vi "Lift_LabVIEW.vi"() -> ()   [LabVIEW 2019]
panel:
  out "Door_Closed":bool
  out "Door_Open":bool
  out "Count":i32
  out "Lift2":bool
  in  "Close":bool
  in  "Open":bool
  out "?":bool
  out "?":bool
  out "?":bool
  out "Target_Pos":i32
  in  "FLOOR_1_DN":bool
  in  "FLOOR_3_UP":bool
  in  "FLOOR_2_DN":bool
  in  "FLOOR_2_UP":bool
  out "Current_Pos":i32
  out "Up/Down":bool
  out "On/Off":bool
  out "Lift":bool
  in  "stop":bool
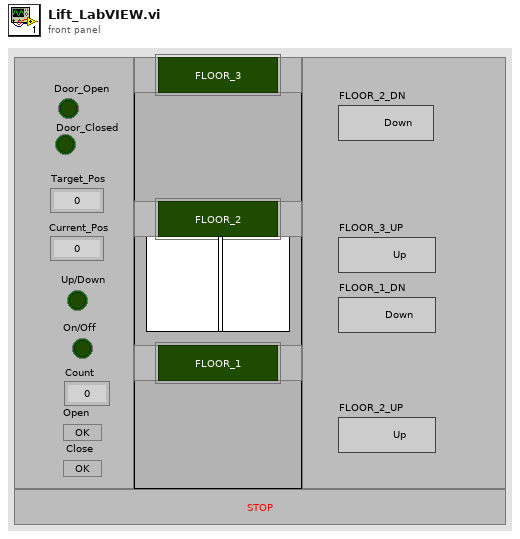
[diagram p1: front panel]
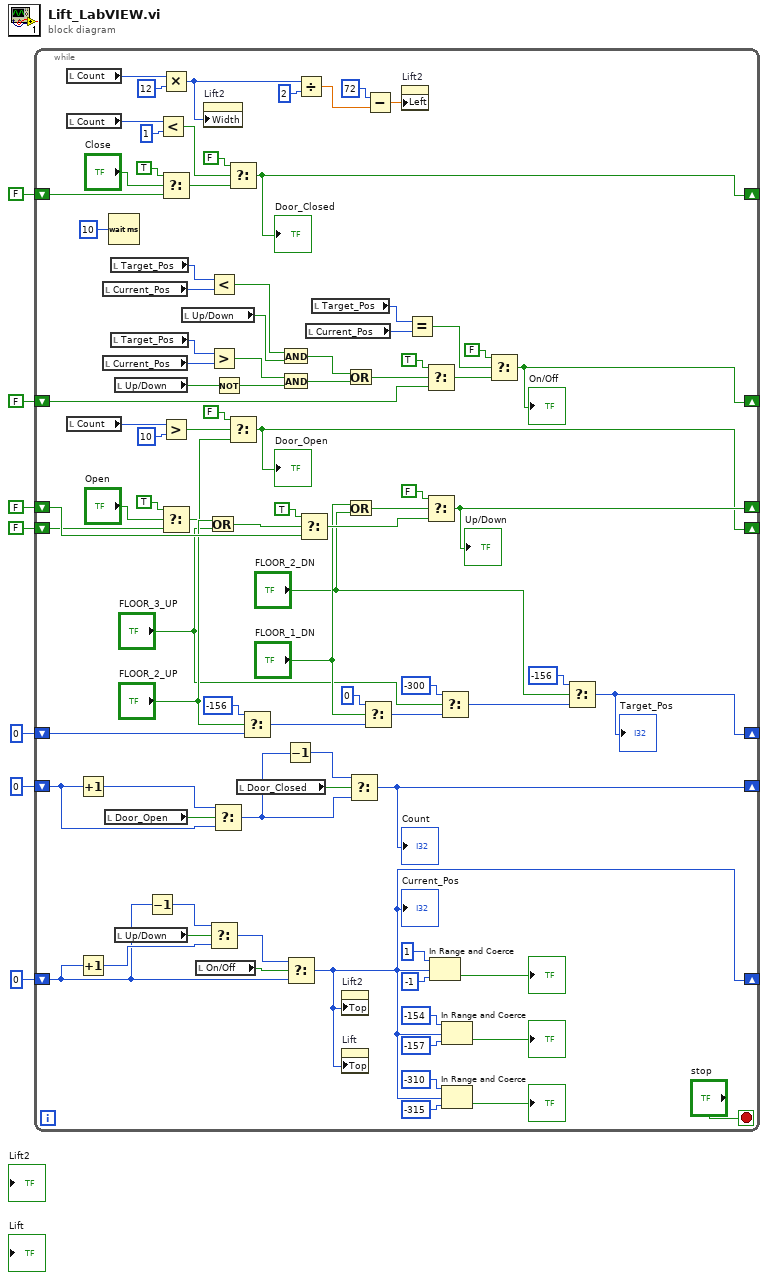
[diagram p0: block diagram]
diagram:
  n1 = while {
    shift-right: [w93] -> _
    shift-left: FALSE -> [w97]
    shift-right: [w8] -> _
    shift-left: 0 -> [w80]
    shift-right: [w84] -> _
    shift-left: FALSE -> [w86]
    shift-right: [w79] -> _
    shift-left: 0 -> [w78]
    shift-right: [w36] -> _
    shift-left: 0 -> [w40]
    shift-right: [w29] -> _
    shift-left: FALSE -> [w32]
    shift-right: [w25] -> _
    shift-left: FALSE -> [w27]
    stop <- "stop" stop-if-true
    n2 = local read "Count"() -> (w15:i32)
    n3 = local read "Count"() -> (w20:i32)
    n4 = local read "Count"() -> (w23:i32)
    n5 = Increment(x=w40) -> (x+1=w38:i32)
    n6 = Increment(x=w80) -> (x+1=w90:i32)
    n7 = local read "Current_Pos"() -> (w64:i32)
    n8 = local read "Current_Pos"() -> (w50:i32)
    n9 = local read "Door_Open"() -> (w17:bool)
    n10 = Wait (ms)(milliseconds to wait=u32 10) -> ()  [unwired: 1 out]
    n11 = local read "Target_Pos"() -> (w65:i32)
    n12 = local read "Target_Pos"() -> (w51:i32)
    n13 = local read "Up/Down"() -> (w54:bool)
    n14 = local read "Up/Down"() -> (w81:bool)
    n15 = Decrement(x=w80) -> (x-1=w91:i32)
    n16 = Less?(x=w20, y=1) -> (x < y?=w18:bool)
    n17 = Multiply(x=w15, y=12) -> (x*y=w12:i32)
    n18 = Select(t=TRUE, s="Close", f=w27) -> (s? t:f=w28:bool)
    n19 = Greater?(x=w23, y=10) -> (0:w21:bool)
    n20 = Select(t=TRUE, s="Open", f=w32) -> (s? t:f=w33:bool)
    n21 = local read "Up/Down"() -> (w62:bool)
    n22 = local read "On/Off"() -> (w88:bool)
    n23 = property on="Lift2" class="Bool (strict)"("Width"=w12) -> ()  [unwired: 2 in, 2 out]
    n24 = Or(x="FLOOR_2_UP", y="FLOOR_3_UP") -> (x .or. y?=w69:bool)
    n25 = Less?(x=w65, y=w64) -> (x < y?=w63:bool)
    n26 = Greater?(x=w51, y=w50) -> (0:w57:bool)
    n27 = Select(t=w91, s=w81, f=w90) -> (s? t:f=w89:i32)
    n28 = Select(t=w38, s=w17, f=w40) -> (s? t:f=w39:i32)
    n29 = Not(x=w54) -> (.not. x?=w55:bool)
    n30 = Select(t=FALSE, s=w18, f=w28) -> (s? t:f=w25:bool)
    "Door_Closed" <- w25
    n31 = Select(t=FALSE, s=w21, f=w33) -> (s? t:f=w29:bool)
    "Door_Open" <- w29
    n32 = local read "Door_Closed"() -> (w16:bool)
    n33 = Select(t=-156, s="FLOOR_2_UP", f=w78) -> (s? t:f=w77:i32)
    n34 = And(x=w63, y=w62) -> (x .and. y?=w61:bool)
    n35 = And(x=w57, y=w55) -> (x .and. y?=w52:bool)
    n36 = Decrement(x=w39) -> (x-1=w37:i32)
    n37 = Select(t=w89, s=w88, f=w80) -> (s? t:f=w8:i32)
    "Current_Pos" <- w8
    n38 = Divide(x=w12, y=2) -> (x/y=w11:dbl)
    n39 = Select(t=TRUE, s=w69, f=w86) -> (s? t:f=w85:bool)
    n40 = local read "Current_Pos"() -> (w59:i32)
    n41 = local read "Target_Pos"() -> (w60:i32)
    n42 = property on="Lift2" class="Bool (strict)"("Top"=w8) -> ()  [unwired: 2 in, 2 out]
    n43 = property on="Lift" class="Bool (strict)"("Top"=w8) -> ()  [unwired: 2 in, 2 out]
    n44 = Or(x=w61, y=w52) -> (x .or. y?=w53:bool)
    n45 = Or(x="FLOOR_1_DN", y="FLOOR_2_DN") -> (x .or. y?=w66:bool)
    n46 = Select(t=w37, s=w16, f=w39) -> (s? t:f=w36:i32)
    "Count" <- w36
    n47 = Select(t=0, s="FLOOR_1_DN", f=w77) -> (s? t:f=w76:i32)
    n48 = Subtract(x=i16 72, y=w11) -> (x-y=w9:dbl)
    n49 = property on="Lift2" class="Bool (strict)"("Left"=w9) -> ()  [unwired: 2 in, 2 out]
    n50 = Equal?(x=w60, y=w59) -> (x = y?=w58:bool)
    n51 = Select(t=TRUE, s=w53, f=w97) -> (s? t:f=w95:bool)
    n52 = Select(t=FALSE, s=w66, f=w85) -> (s? t:f=w84:bool)
    "Up/Down" <- w84
    n53 = In Range and Coerce(upper limit=1, x=w8, lower limit=-1) -> (In Range?=→"?":bool)  [unwired: 1 out]
    n54 = Select(t=-300, s="FLOOR_3_UP", f=w76) -> (s? t:f=w75:i32)
    n55 = In Range and Coerce(upper limit=-154, x=w8, lower limit=-157) -> (In Range?=→"?":bool)  [unwired: 1 out]
    n56 = In Range and Coerce(upper limit=-310, x=w8, lower limit=-315) -> (In Range?=→"?":bool)  [unwired: 1 out]
    n57 = Select(t=FALSE, s=w58, f=w95) -> (s? t:f=w93:bool)
    "On/Off" <- w93
    n58 = Select(t=-156, s="FLOOR_2_DN", f=w75) -> (s? t:f=w79:i32)
    "Target_Pos" <- w79
  }
